vi "gu_create_file.vi"(8 "error in":errorcluster, 11 "Encoded String":T1) -> (0 "error out":errorcluster)   [LabVIEW 2020, in "G-Unicode.lvlib"]
uses:
  G-Unicode.lvlib
  Types/Encoded UTF-8 String.ctl
  lib/g_unicode_32.dll
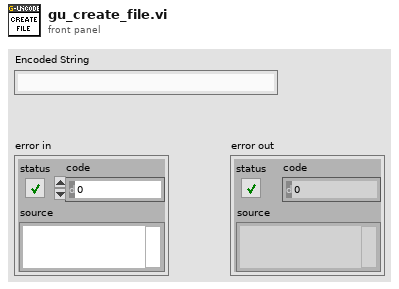
[diagram p1: front panel]
types:
  T1 = typedef "G-Unicode.lvlib/Encoded UTF-8 String.ctl" = string
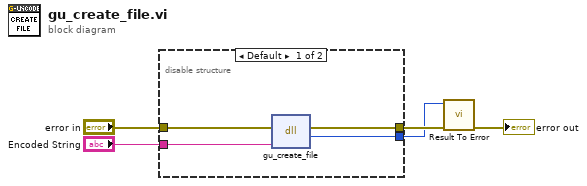
[diagram p0: block diagram]
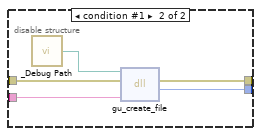
[diagram p2: hidden frame]
diagram:
  n1 = disable-structure shown="Default" {
    disable-tunnel: [w9 w14] -> w5
    disable-tunnel: [w6 w13] -> w1
    disable-tunnel: "Encoded String" -> [w8 w12]
    disable-tunnel: "error in" -> [w7 w11]
    frame condition #0 (active) {
      n2 = dll-call lib="C:/github/dataflowg/g-unicode/src/LabVIEW/G-Unicode/lib/g_unicode_*.*" fn="gu_create_file"(error in=w7, "utf8_path"=w8) -> (error out=w9:errorcluster, "result"=w6:i32)  [unwired: 3 in, 1 out]
    }
    frame condition #1 {
      n3 = call "_Debug Path.vi"() -> ("Debug Path"=w10:path)
      n4 = dll-call lib="?" fn="gu_create_file"(path in=w10, error in=w11, "utf8_path"=w12) -> (error out=w14:errorcluster, "result"=w13:i32)  [unwired: 2 in, 1 out]
    }
  }
  n5 = call "Result To Error.vi"("error in (no error)"=w5, "Result Code"=w1) -> ("error out"=→"error out":errorcluster)  [unwired: 9 in]
